vi "Orientation Measurements.vi"(8 "Disturbance length (samples)":i32, 9 "Disturbance cluster":T2={"Disturbance T/F"=FALSE, "Disturbance\nAmplitude [deg]"=1.0} {"Disturbance\nAmplitude [deg]" format="%#_13g"}, 10 "error in (no error)":errorcluster, 11 "FPGA Interface":refnum<k20>) -> (1 "Position data":T1, 2 "error out":errorcluster, 3 "FPGA Interface Out":refnum<k20>)   [LabVIEW 2016]
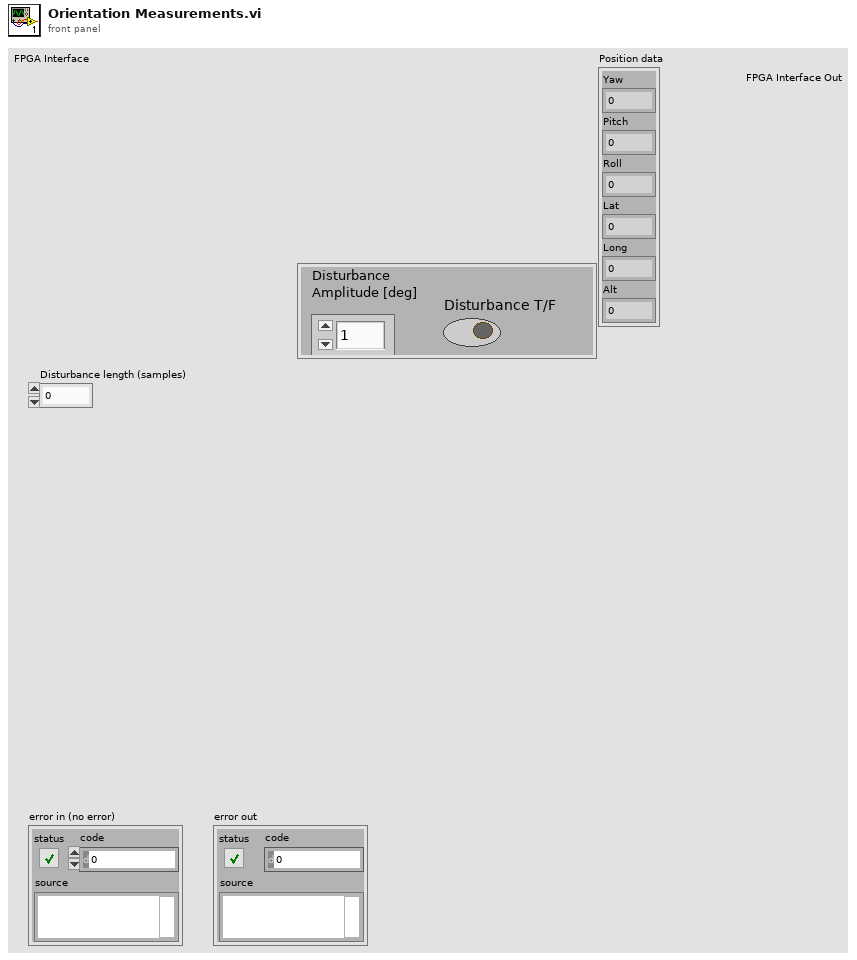
[diagram p1: front panel]
types:
  T1 = cluster{"Yaw":sgl, "Pitch":sgl, "Roll":sgl, "Lat":dbl, "Long":dbl, "Alt":dbl}
  T2 = cluster{"Disturbance T/F":bool, "Disturbance\nAmplitude [deg]":dbl}
  T3 = typedef "INS Data.ctl" = cluster{"Yaw":sgl, "Pitch":sgl, "Roll":sgl, "Lat":dbl, "Long":dbl, "Alt":dbl, "North":dbl, "East":dbl, "Down":dbl, "PosU":dbl, "VelU":dbl}
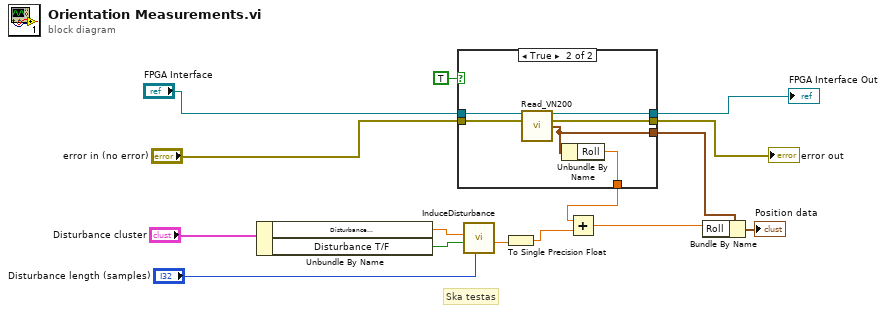
[diagram p0: block diagram]
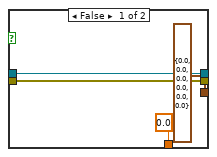
[diagram p2: hidden frame]
diagram:
  # "Ska testas"
  n1 = Unbundle By Name("Disturbance cluster") -> ("Disturbance\nAmplitude [deg]"=w13:dbl, "Disturbance T/F"=w12:bool)
  n2 = case shown="True" TRUE {
    tunnel: "error in (no error)" -> [w18 w25]
    tunnel: [w18 w24] -> w10
    tunnel: [sgl 0.0 ("Roll") w23] -> w9
    tunnel: [T1 {"Yaw"=0.0, "Pitch"=0.0, "Roll"=0.0, "Lat"=0.0, "Long"=0.0, "Alt"=0.0} ("Position Data") w22] -> w6
    tunnel: "FPGA Interface" -> [w19 w21]
    tunnel: [w19 w20] -> w2
    frame False {
    }
    frame True {
      n3 = call "Read_VN200.vi"("FPGA Interface"=w21, "error in"=w25) -> ("FPGA Interface Out"=w20:refnum<k20>, "error out"=w24:errorcluster, "Position Data"=w22:T3)  [unwired: 11 in]
      n4 = Unbundle By Name(w22) -> ("Roll"=w23:sgl)
    }
  }
  "error out" <- w10
  "FPGA Interface Out" <- w2
  n5 = call "InduceDisturbance.vi"("Disturbance length\n (number of iterations)"="Disturbance length (samples)", "Disturbance"=w12, "Disturbance\nAmplitude [deg]"=w13) -> ("Disturbance\nAmplitude"=w8:dbl)  [unwired: 7 in, 1 out]
  n6 = To Single Precision Float(number=w8) -> (single precision float=w7:sgl)
  n7 = Add(x=w9, y=w7) -> (x+y=w5:sgl)
  n8 = Bundle By Name(cluster=w6, "Roll"=w5) -> (→"Position data":T3)
